vi "Create.vi"(8 "error in (no error)":errorcluster, 9 "CS Active Low":bool, 10 "GPIO":T1=-1) -> (0 "error out":errorcluster, 3 "SPI CS out":refnum<class "SPI CS.lvclass">)   [LabVIEW 2024, in "CTI.lvlib" / "SPI CS.lvclass"]
uses:
  SPI CS.lvclass
  GPIO Number.ctl
  SPI CS.lvclass/SPI CS.ctl
  CTI.lvlib
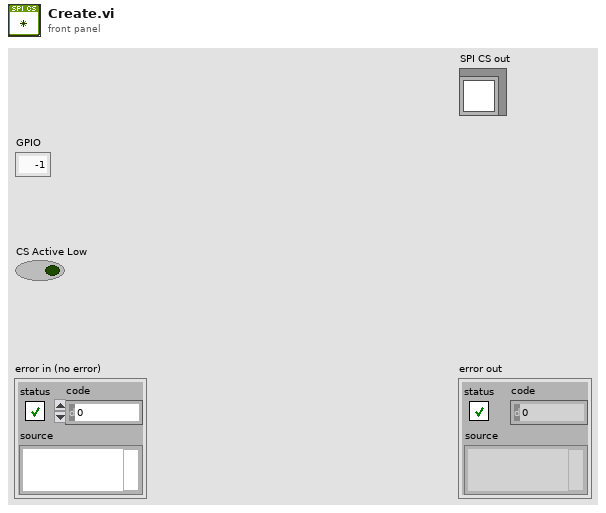
[diagram p1: front panel]
types:
  T1 = typedef "CTI.lvlib/GPIO Number.ctl" = i8
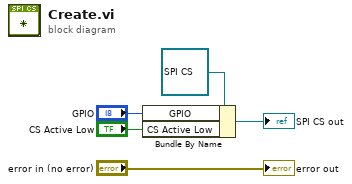
[diagram p0: block diagram]
diagram:
  n1 = Bundle By Name(cluster=refnum<class "SPI CS.lvclass"> refnum ("SPI CS in"), "GPIO"="GPIO", "CS Active Low"="CS Active Low") -> (→"SPI CS out":refnum<class "SPI CS.lvclass">)
  "error out" <- "error in (no error)"
